vi "Testhold_ClusterToString_Array.vi"(8 "SLG_Cluster4":T1, 9 "SLG_Cluster3":T1, 10 "SLG_Cluster2":T1, 11 "SLG_Cluster":T1) -> (2 "String_Array":string[](array[string]))   [LabVIEW 2019]
uses:
  Test_load.ctl
  TEST.lvclass
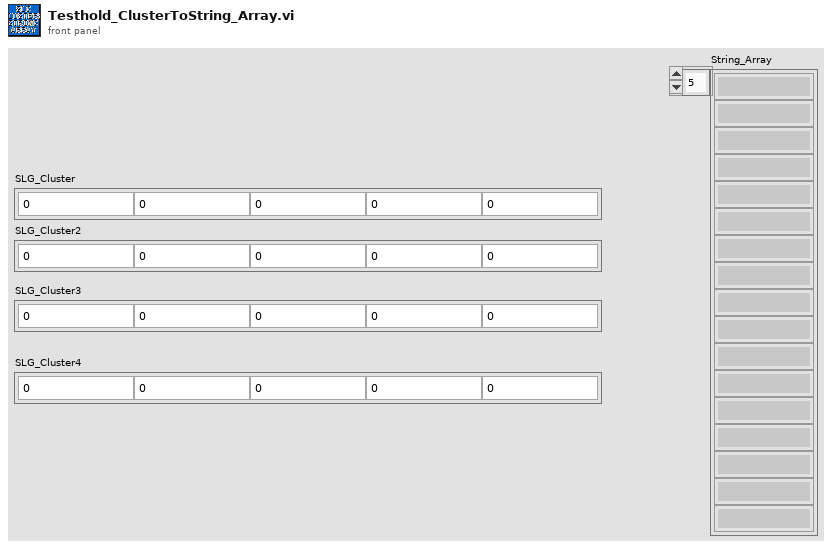
[diagram p1: front panel]
types:
  T1 = typedef "TEST.lvclass/Test_load.ctl" = cluster{"TEST1":sgl, "TEST2":sgl, "TEST3":sgl, "DEV":sgl, "INACC":sgl}
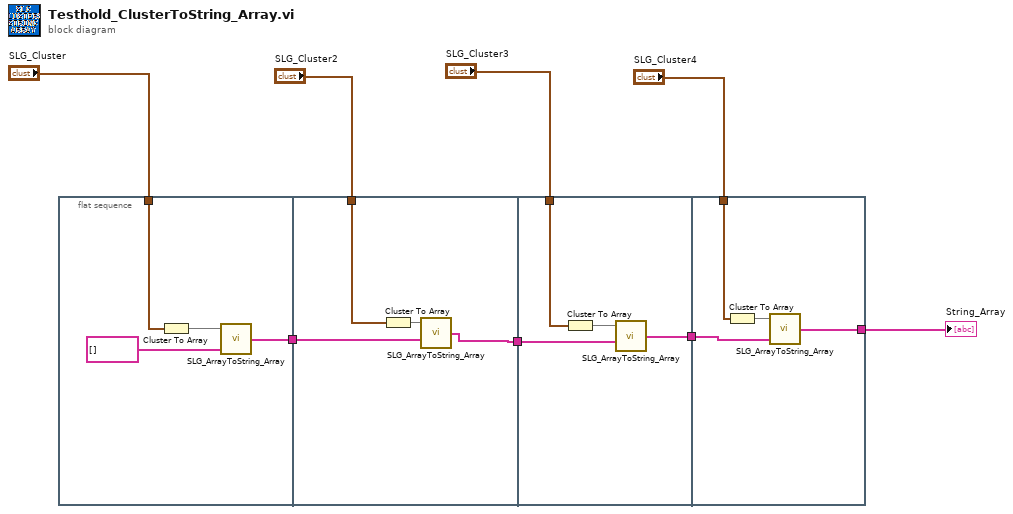
[diagram p0: block diagram]
diagram:
  n1 = flat-sequence {
    tunnel: [w10] -> w8
    tunnel: "SLG_Cluster" -> [w12]
    tunnel: w8 -> [w15]
    tunnel: [w13] -> w7
    tunnel: "SLG_Cluster2" -> [w16]
    tunnel: w7 -> [w19]
    tunnel: "SLG_Cluster3" -> [w20]
    tunnel: [w17] -> w2
    tunnel: "SLG_Cluster4" -> [w24]
    tunnel: w2 -> [w23]
    tunnel: [w21] -> w1
    frame #0 {
      n2 = Cluster To Array(cluster=w12) -> (array=w9:sgl[])
      n3 = call "SLG_ArrayToString_Array.vi"("OrArray"=string[] [], "SLG_Array"=w9) -> ("StringArray"=w10:string[])  [unwired: 1 in]
    }
    frame #1 {
      n4 = Cluster To Array(cluster=w16) -> (array=w14:sgl[])
      n5 = call "SLG_ArrayToString_Array.vi"("OrArray"=w15, "SLG_Array"=w14) -> ("StringArray"=w13:string[])  [unwired: 1 in]
    }
    frame #2 {
      n6 = Cluster To Array(cluster=w20) -> (array=w18:sgl[])
      n7 = call "SLG_ArrayToString_Array.vi"("OrArray"=w19, "SLG_Array"=w18) -> ("StringArray"=w17:string[])  [unwired: 1 in]
    }
    frame #3 {
      n8 = Cluster To Array(cluster=w24) -> (array=w22:sgl[])
      n9 = call "SLG_ArrayToString_Array.vi"("OrArray"=w23, "SLG_Array"=w22) -> ("StringArray"=w21:string[])  [unwired: 1 in]
    }
  }
  "String_Array" <- w1
